vi "lectVectCentergravity.vi"() -> ()   [LabVIEW 2020]
panel:
  out "decimated array 3":sgl[](graph)
  out "decimated array 2":sgl[](graph)
  in  "Path":path
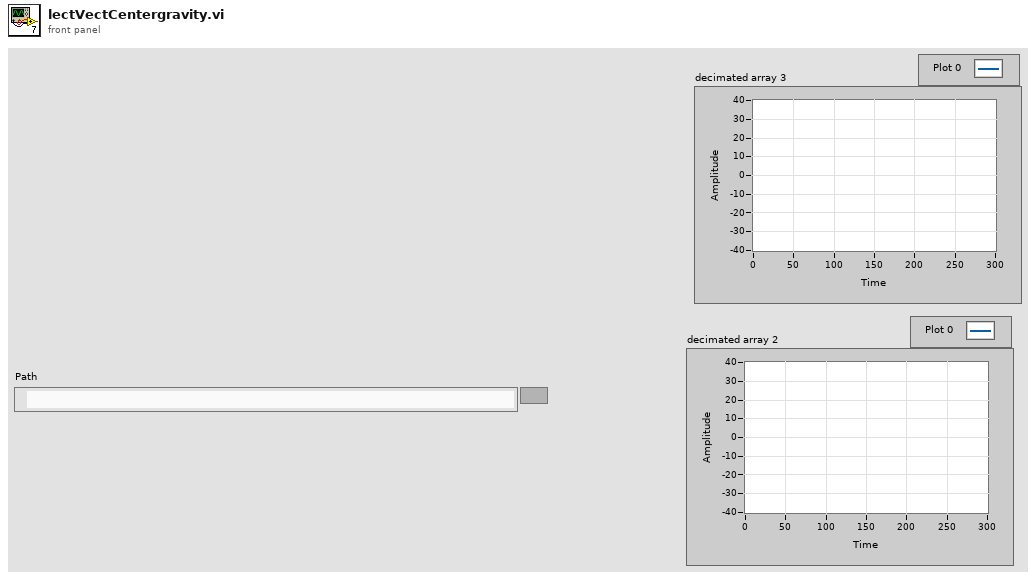
[diagram p1: front panel]
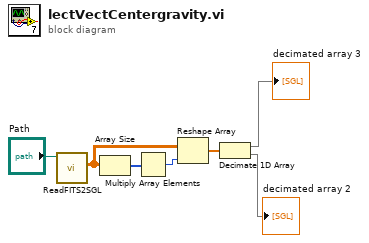
[diagram p0: block diagram]
diagram:
  n1 = call "ReadFITS2SGL.vi"("Path"="Path") -> ("Tableau2DSGL"=w4:sgl[][])  [unwired: 7 in, 3 out]
  n2 = Array Size(array=w4) -> (size(s)=w7:i32[])
  n3 = Multiply Array Elements(1:w7) -> (0:w6:i32)
  n4 = Reshape Array(w4, w6) -> (w5:sgl[])
  n5 = Decimate 1D Array(w5) -> (→"decimated array 3":sgl[], →"decimated array 2":sgl[])
